vi "Vibration main_exercise.vi"() -> ()   [LabVIEW 2012]
uses:
  <vilib>/measure/maspectr.llb/Power Spectrum and PSD Export Mode.ctl
  <vilib>/measure/NI_MAPro.lvlib
  <vilib>/Analysis/4window.llb/windowTd.ctl
  <vilib>/Analysis/NI_AALPro.lvlib
panel:
  out "Detected Amplitude":dbl
  out "Fan Warning":bool
  in  "Max Vib Level":dbl=0.03
  out "Detected Tone":dbl
  in  "Fan Speed Channel":tag="Voltage_out/ao1"
  in  "Tab Control":enum32{"LabVIEW PS", "MathScript PS"}(tab)
  out "LabVIEW PS":cluster{"f0":dbl, "df":dbl, "magnitude":dbl[]}(graph)={"f0"=0.0, "df"=10.240000000000004, "magnitude"=[]}
  out "MathScript PS":cluster{dbl, "df":dbl, "freq":dbl[]}(graph)={0.0, "df"=10.240000000000004, "freq"=[]}
  in  "Fan Speed":dbl(knob) scale=0.0..10.0
  out "Time Domain":waveform(dbl)(graph)={"t0"=timestamp(3438622544.0521445 s since 1904-01-01), "dt"=9.765624999999998e-05, "Y"=array[1000 elements], "attributes"=variant("NI_ChannelName"=variant(string "Sound_Vibration/ai0"), "NI_UnitDescription"=variant(string "g"), "NI_dBReference"=variant(dbl 1.0))}
  in  "Sample Rate":dbl=10000.0
  in  "Samples Per Channel":i32=1000
  in  "Stop Button":bool
  in  "Vibration Channel":tag="Sound_Vibration/ai0"
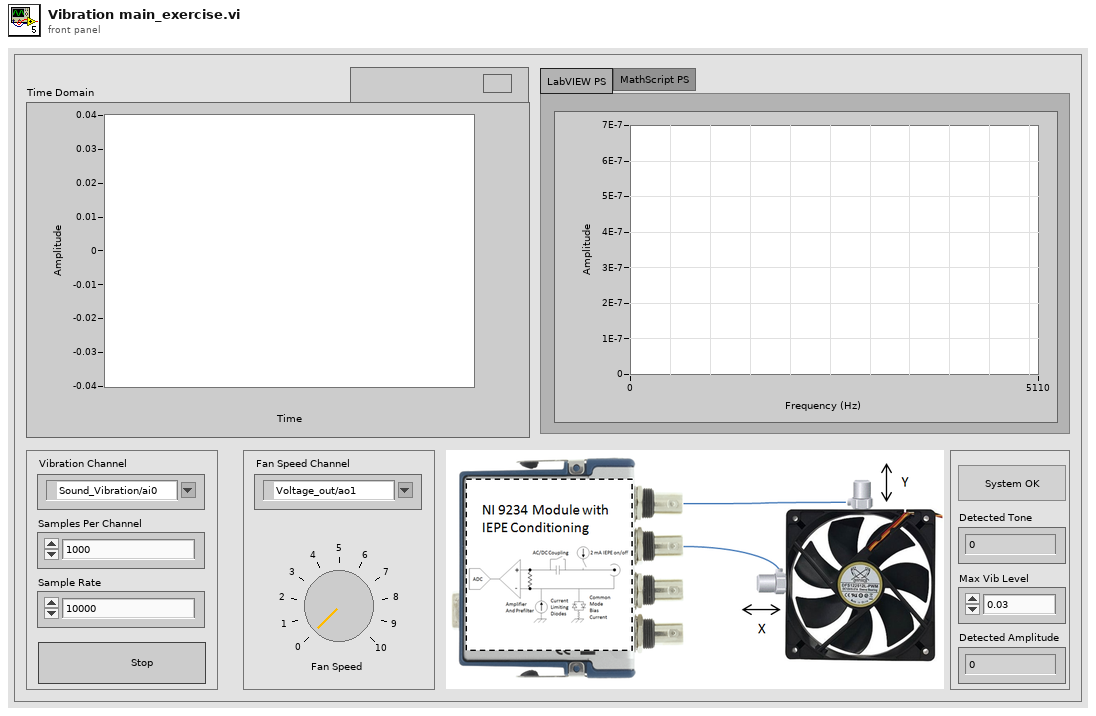
[diagram p1: front panel]
types:
  T1 = typedef "NI_AALPro.lvlib/windowTd.ctl" = u32
  T2 = typedef "NI_MAPro.lvlib/Power Spectrum and PSD Export Mode.ctl" = u16
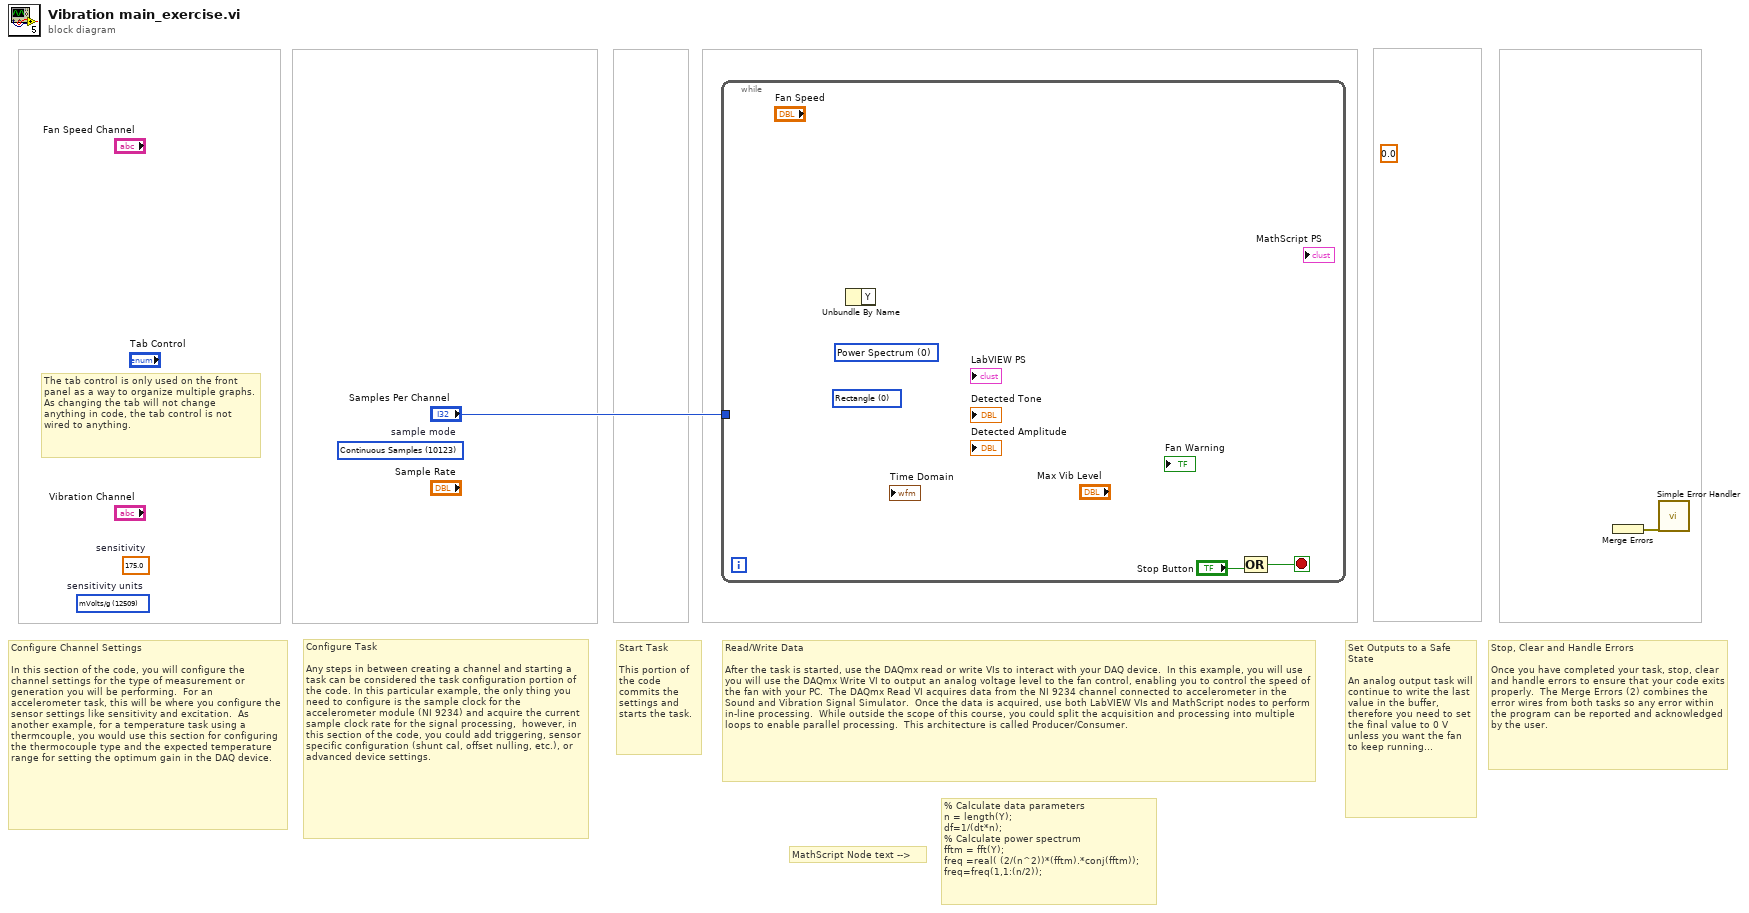
[diagram p0: block diagram]
diagram:
  (unwired) 0.0 ("data")
  (unwired) 12509 items=["mVolts/g"=12509, "Volts/g"=12510]  # sensitivity units
  (unwired) 175.0  # sensitivity
  (unwired) 10123 items=["Finite Samples"=10178, "Continuous Samples"=10123, "Hardware Timed Single Point"=12522]  # sample mode
  # "MathScript Node text -->"
  # "% Calculate data parameters\nn = length(Y); \ndf=1/(dt*n);\n% Calculate power spectrum\nfftm = fft(Y);\nfreq =real( (2/(n^2))*(fftm).*conj(fftm));\nfreq=freq(1,1:(n/2));"
  # "The tab control is only used on the front panel as a way to organize multiple graphs.  As changing the tab will not change anything in code, the tab control is not wired to anything."
  # "Set Outputs to a Safe State\n\nAn analog output task will continue to write the last value in the buffer, therefore you need to set the final value to 0 V unless you want the fan to keep running..."
  # "Stop, Clear and Handle Errors\n\nOnce you have completed your task, stop, clear and handle errors to ensure that your code exits properly.  The Merge Errors (2) combines the error wires from both tasks so any error within the program can be reported and acknowledged by the user."
  # "Read/Write Data\n\nAfter the task is started, use the DAQmx read or write VIs to interact with your DAQ device.  In this example, you will use you will use the DAQmx Write VI to output an analog voltage level to the fan control, enabling you to control the speed of the fan with your PC.  The DAQmx Read VI acquires data from the NI 9234 channel connected to accelerometer in the Sound and Vibration Signal Simulator.  Once the data is acquired, use both LabVIEW VIs and MathScript nodes to perform in-line processing.  While outside the scope of this course, you could split the acquisition and processing into multiple loops to enable parallel processing.  This architecture is called Producer/Consumer."
  # "Start Task\n\nThis portion of the code commits the settings and starts the task."
  # "Configure Task\n\nAny steps in between creating a channel and starting a task can be considered the task configuration portion of the code. In this particular example, the only thing you need to configure is the sample clock for the accelerometer module (NI 9234) and acquire the current sample clock rate for the signal processing,  however, in this section of the code, you could add triggering, sensor specific configuration (shunt cal, offset nulling, etc.), or advanced device settings."
  # "Configure Channel Settings\n\nIn this section of the code, you will configure the channel settings for the type of measurement or generation you will be performing.  For an accelerometer task, this will be where you configure the sensor settings like sensitivity and excitation.  As another example, for a temperature task using a thermcouple, you would use this section for configuring  the thermocouple type and the expected temperature range for setting the optimum gain in the DAQ device."
  n1 = while {
    tunnel: "Samples Per Channel" -> [_]
    stop <- w4 stop-if-true
    (unwired) T1 0 items=["Rectangle"=0, "Hanning"=1, "Hamming"=2, "Blackman-Harris"=3, "Exact Blackman"=4, "Blackman"=5, "Flat Top"=6, "4 Term B-Harris "=7, "7 Term B-Harris"=8, "Low Sidelobe"=9, "Blackman Nuttall"=11, "Triangle"=30, "Bartlett-Hanning"=31, "Bohman"=32, "Parzen"=33, "Welch"=34, "Kaiser"=60, "Dolph-Chebyshev"=61, "Gaussian"=62] ("window")
    (unwired) T2 0 items=["Power Spectrum", "Power Spectral Density"] ("export mode")
    n2 = Unbundle By Name() -> ()  [unwired: 1 in, 1 out]
    n3 = Compound Arithmetic op=OR("Stop Button") -> (w4:bool)  [unwired: 1 in]
  }
  n4 = Merge Errors() -> (w2:errorcluster)  [unwired: 1 in]
  n5 = call <vilib>:"Simple Error Handler.vi"("error in (no error)"=w2) -> ()  [unwired: 4 in, 5 out]
